vi "Order Tracking (Analog Tach).vi"(0 "scaled signal [EU]":waveform(dbl)={"t0"=timestamp(0 s since 1904-01-01), "dt"=0.0, "Y"=[]}, 4 "analog tach signal":waveform(dbl)={"t0"=timestamp(0 s since 1904-01-01), "dt"=0.0, "Y"=[]}, 5 "pulse/revolution (1)":dbl=1.0 format="%.2f", 6 "orders (1.0)":dbl[](array[numeric])=[1.0] format="%.2f", 7 "averaging type":enum16{"Linear", "Exponential"}(ring), 8 "bandwidth":T5={"bandwidth value"=0.5, "bandwidth unit"=enum."Order"} {"bandwidth value" min=0.0 format="%.2f"}, 9 "averaging parameters":T2={"exponential mode"=enum."Fast", "time constant [ms]"=125.0, "decimating factor"=1} {"decimating factor" min=1 step=1; "time constant [ms]" format="%.2f"}, 10 "window info":T4={"window type"=3, "window length"=2048} {"window type" items=["None"=0, "Hanning"=1, "Hamming"=2, "Blackman-Harris"=3, "Exact Blackman"=4, "Blackman"=5, "Flat Top"=6, "4 Term B-Harris"=7, "7 Term B-Harris"=8, "Low Sidelobe"=9, "Gaussian"=62]; "window length" min=0}, 11 "view mode":enum16{"Power", "Amplitude", "dB"}(ring)=enum."Amplitude") -> (13 "speed profile":T1 {"speed [RPM]" format="%.2f"; "time [s]" format="%.2f"}, 14 "order waveforms [EU]":waveform(dbl)[](array[waveform]), 15 "waveform unit":string, 17 "orders magnitudes":waveform(dbl)[](array[waveform]), 18 "magnitudes vs. rpm":T3(array[cluster]) {"magnitude" format="%.2f"; "delta rpm" format="%.2f"; "rpm 0" format="%.2f"}, 19 "unit label":string)   [LabVIEW 2017]
doc: "Extracts designated orders from <B>scaled signal</B> using <B>analog tach signal</B> and computes magnitudes for the designated orders."
uses:
  <vilib>/addons/Sound and Vibration/Order Analysis/Ref Gabor Order Tracking/Mask Bandwidth.ctl
  <vilib>/addons/Sound and Vibration/Order Analysis/Ref Gabor Order Tracking/window information.ctl
  <vilib>/addons/Sound and Vibration/Order Analysis/Tach Process/SubVIs/speed profile.ctl
  <vilib>/addons/Sound and Vibration/Order Analysis/Tach Process/SoundVib_TachProcess.lvlib
  <vilib>/addons/Sound and Vibration/Order Analysis/Gabor Order Tracking/SoundVib_Gabor.lvlib
panel:
  # "Order Tracking (Analog Tach)"
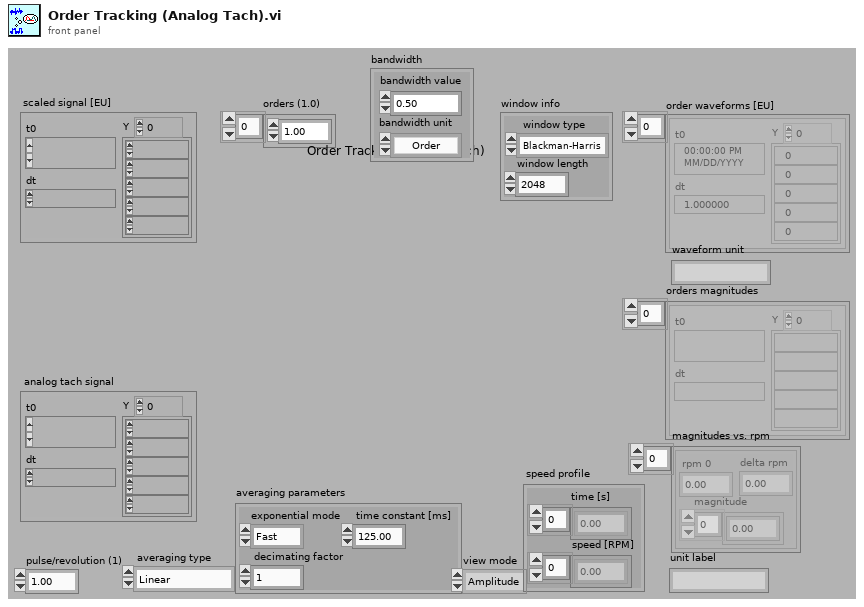
[diagram p1: front panel]
types:
  T1 = typedef "SoundVib_TachProcess.lvlib/speed profile.ctl" = cluster{"time [s]":dbl[], "speed [RPM]":dbl[]}
  T2 = cluster{"exponential mode":enum16{"Slow", "Fast", "Impulse", "Custom"}, "time constant [ms]":dbl, "decimating factor":i32}
  T3 = cluster{"rpm 0":dbl, "delta rpm":dbl, "magnitude":dbl[]}[]
  T4 = typedef "SoundVib_Gabor.lvlib/window information.ctl" = cluster{"window type":u32, "window length":i32}
  T5 = typedef "SoundVib_Gabor.lvlib/Mask Bandwidth.ctl" = cluster{"bandwidth value":dbl, "bandwidth unit":enum16{"Order", "Hz"}}
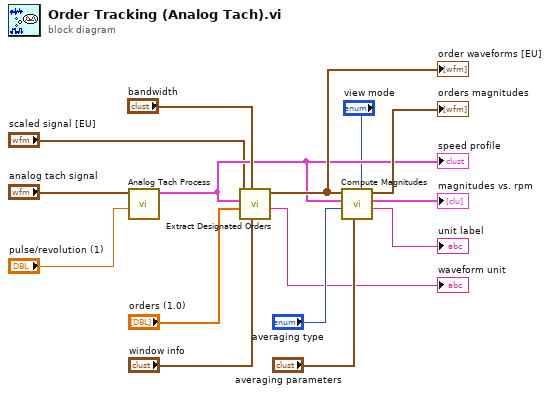
[diagram p0: block diagram]
diagram:
  n1 = call <vilib>:"Analog Tach Process.vi"("pulse/revolution (1)"="pulse/revolution (1)", "analog tach signal"="analog tach signal") -> ("speed profile"=w7:T1)  [unwired: 7 in, 2 out]
  "speed profile" <- w7
  n2 = call <vilib>:"Extract Designated Orders.vi"("window info"="window info", "bandwidth"="bandwidth", "orders (1.0)"="orders (1.0)", "speed profile"=w7, "scaled signal [EU]"="scaled signal [EU]") -> ("unit label"=→"waveform unit":string, "order waveforms [EU]"=w9:waveform(dbl)[])  [unwired: 3 in, 2 out]
  "order waveforms [EU]" <- w9
  n3 = call <vilib>:"Compute Magnitudes.vi"("view mode"="view mode", "averaging parameters"="averaging parameters", "averaging type"="averaging type", "speed profile"=w7, "order waveforms [EU]"=w9) -> ("unit label"=→"unit label":string, "magnitudes vs. rpm"=→"magnitudes vs. rpm":T3, "orders magnitudes"=→"orders magnitudes":waveform(dbl)[])  [unwired: 4 in]
